vi "Y坐标上下翻转.vi"(10 "数组输入":cluster{"X":dbl, "Y":dbl}[](array[cluster]), 11 "数值":dbl) -> (3 "数组输出":cluster{"X":dbl, "Y":dbl}[](array[cluster]))   [LabVIEW 2014]
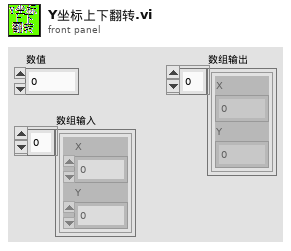
[diagram p1: front panel]
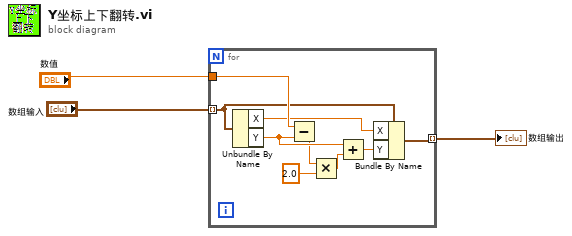
[diagram p0: block diagram]
diagram:
  n1 = for {
    tunnel: "数组输入" -> [w10] mode=indexing
    tunnel: "数值" -> [w12]
    tunnel: [w8] -> w2 mode=indexing
    n2 = Unbundle By Name(w10) -> ("X"=w9:dbl, "Y"=w11:dbl)
    n3 = Subtract(x=w12, y=w11) -> (x-y=w5:dbl)
    n4 = Multiply(x=w5, y=2.0) -> (x*y=w4:dbl)
    n5 = Add(x=w11, y=w4) -> (x+y=w6:dbl)
    n6 = Bundle By Name(cluster=w10, "X"=w9, "Y"=w6) -> (w8:cluster{"X":dbl, "Y":dbl})
  }
  "数组输出" <- w2
